vi "DD_OpenRef_TS_Step.vi"(0 "Engine Reference":refnum<k7>, 1 "Precondition":string, 5 "Sequence File Ref":refnum<k7>, 7 "Step Name":string="Open DD", 9 "Requirement":string, 11 "error in":errorcluster, 12 "index":i32, 13 "Attended?":bool) -> (4 "Engine reference(out)":refnum<k7>, 6 "Sequence File Ref(out)":refnum<k7>, 15 "error out":errorcluster)   [LabVIEW 2010]
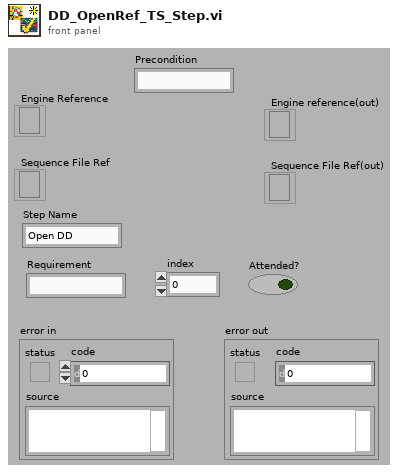
[diagram p1: front panel]
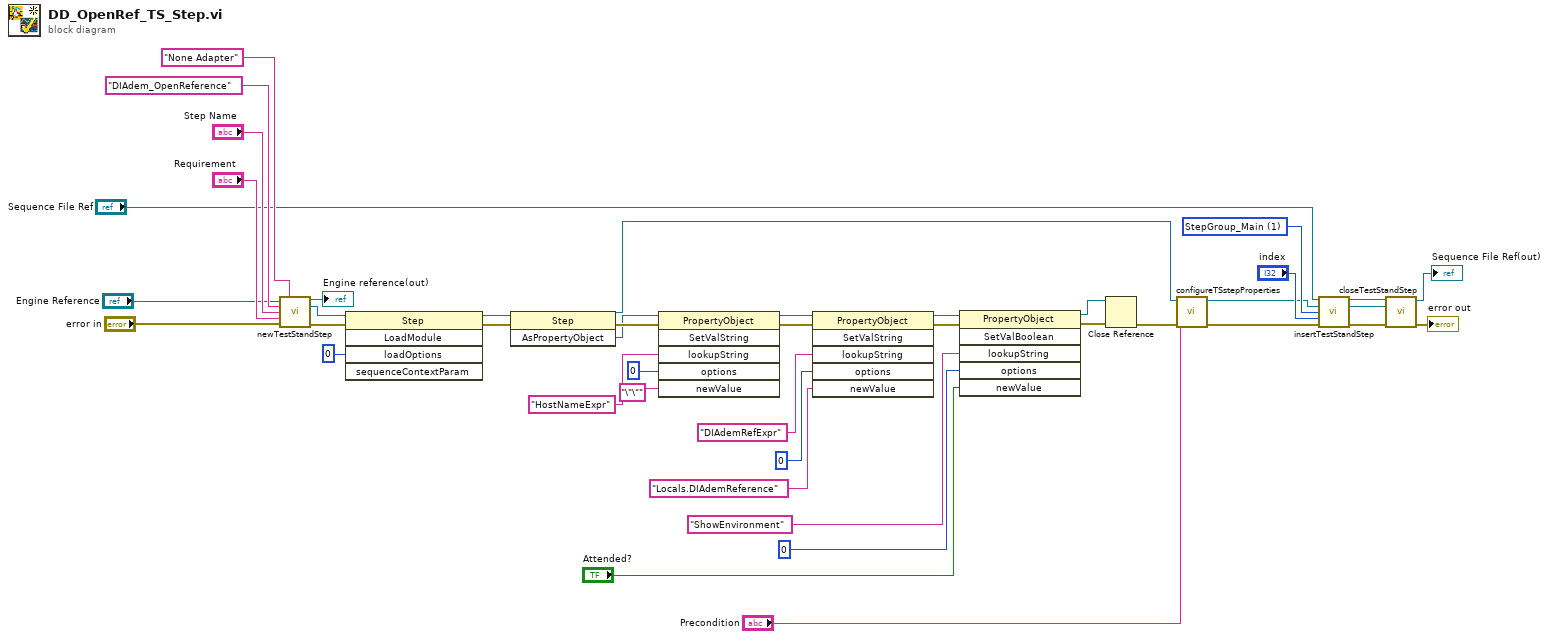
[diagram p0: block diagram]
diagram:
  w27 = 1 items=["StepGroup_Setup", "StepGroup_Main", "StepGroup_Cleanup"] ("Step Group")
  n1 = call "newTestStandStep.vi"("Engine reference"="Engine Reference", "adapterKeyNameVal"="None Adapter", "stepType"="DIAdem_OpenReference", "Step Name"="Step Name", "Requirement"="Requirement", "error in"="error in") -> ("Engine reference(out)"=→"Engine reference(out)":refnum<k7>, "NewStep (out)"=w24:refnum<k7>, "error out"=w25:errorcluster)  [unwired: 7 in]
  n2 = invoke class="Step" method="LoadModule"(reference=w24, error in=w25, "loadOptions"=0) -> (reference out=w31:refnum<k7>, error out=w32:errorcluster)  [unwired: 2 in, 3 out]
  n3 = invoke class="Step" method="AsPropertyObject"(reference=w31, error in=w32) -> (reference out=w3:refnum<k7>, error out=w34:errorcluster, "AsPropertyObject"=w33:refnum<k7>)  [unwired: 1 in]
  n4 = invoke class="PropertyObject" method="SetValString"(reference=w33, error in=w34, "lookupString"="HostNameExpr", "options"=0, "newValue"="\"\"") -> (reference out=w38:refnum<k7>, error out=w39:errorcluster)  [unwired: 1 in, 4 out]
  n5 = invoke class="PropertyObject" method="SetValString"(reference=w38, error in=w39, "lookupString"="DIAdemRefExpr", "options"=0, "newValue"="Locals.DIAdemReference") -> (reference out=w15:refnum<k7>, error out=w14:errorcluster)  [unwired: 1 in, 4 out]
  n6 = invoke class="PropertyObject" method="SetValBoolean"(reference=w15, error in=w14, "lookupString"="ShowEnvironment", "options"=0, "newValue"="Attended?") -> (reference out=w6:refnum<k7>, error out=w7:errorcluster)  [unwired: 1 in, 4 out]
  n7 = Close Reference(reference=w6, error in (no error)=w7) -> (error out=w5:errorcluster)
  n8 = call "configureTSstepProperties.vi"("error in"=w5, "Precondition"="Precondition", "NewStep (in)"=w3) -> ("error out"=w4:errorcluster, "NewStep (out)"=w2:refnum<k7>)  [unwired: 7 in]
  n9 = call "insertTestStandStep.vi"("Sequence File Ref"="Sequence File Ref", "Step to insert"=w2, "Step Group"=w27, "index"="index", "error out"=w4) -> ("Sequence File Ref(out)"=w17:refnum<k7>, "Step to insert (out)"=w18:refnum<k7>, "error out"=w28:errorcluster)  [unwired: 8 in]
  n10 = call "closeTestStandStep.vi"("error in"=w28, "NewStep"=w18, "Sequence File Ref"=w17) -> ("error out"=→"error out":errorcluster, "Sequence File Ref(out)"=→"Sequence File Ref(out)":refnum<k7>)  [unwired: 7 in]
